vi "next_img_name.vi"(8 "error in (no error)":errorcluster, 11 "name in":string) -> (0 "error out":errorcluster, 3 "name out":string)   [LabVIEW 2024, in "Vision.lvlib"]
uses:
  Vision.lvlib
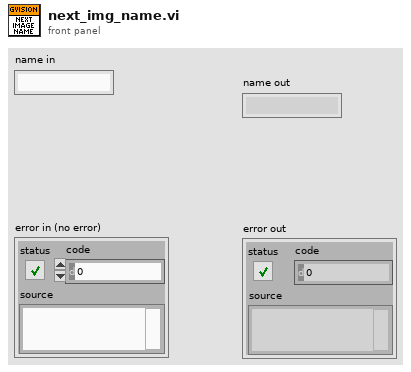
[diagram p1: front panel]
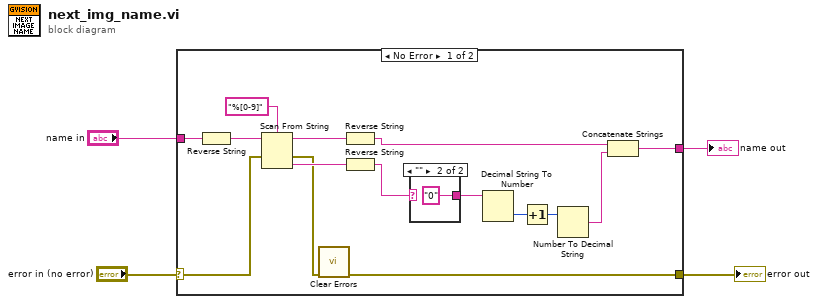
[diagram p0: block diagram]
diagram:
  n1 = case shown="No Error" "error in (no error)" {
    selector: "error in (no error)" -> [w6 w22]
    tunnel: [w5 w22] -> w3
    tunnel: "name in" -> [w19 _]
    tunnel: [w8 _] -> w1
    frame No Error {
      n2 = Reverse String(1:w19) -> (0:w18:string)
      n3 = Scan From String(format string="%[0-9]", input string=w18, error in=w6) -> (remaining string=w16:string, error out=w7:errorcluster, output 1=w15:string)  [unwired: 2 in, 1 out]
      n4 = call <vilib>:"Clear Errors.vi"("error in (no error)"=w7) -> ("error out"=w5:errorcluster)  [unwired: 5 in, 1 out]
      n5 = Reverse String(1:w16) -> (0:w10:string)
      n6 = Reverse String(1:w15) -> (0:w14:string)
      n7 = case shown="\"\"" w14 {
        selector: w14 -> [w20 _]
        tunnel: [w20 "0"] -> w13
        frame Default {
        }
        frame "" {
        }
      }
      n8 = Decimal String To Number(string=w13) -> (number=w12:i32)  [unwired: 2 in, 1 out]
      n9 = Increment(x=w12) -> (x+1=w11:i32)
      n10 = Number To Decimal String(number=w11) -> (decimal integer string=w9:string)  [unwired: 1 in]
      n11 = Concatenate Strings(w10, w9) -> (w8:string)
    }
    frame Error {
    }
  }
  "error out" <- w3
  "name out" <- w1
